vi "Get Environment Variable.vi"(7 "Target (Process)":T1 items=["Process", "User", "Machine"], 8 "Error In":errorcluster, 11 "Name":string) -> (0 "Error Out":errorcluster, 3 "Value":string)   [LabVIEW 2019, in "SLL Environment Variable.lvlib"]
doc: "Get <B>Value</B> of environment variable from <B>Target</B> environment."
uses:
  SLL Environment Variable.lvlib
  _Typedef/Target Environment Enum.ctl
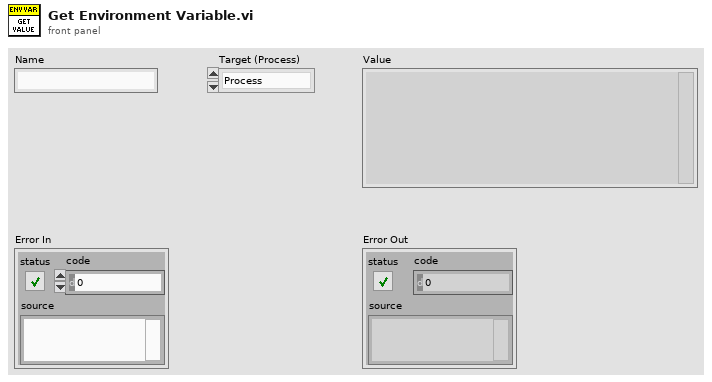
[diagram p1: front panel]
types:
  T1 = typedef "SLL Environment Variable.lvlib/Target Environment Enum.ctl" = i32
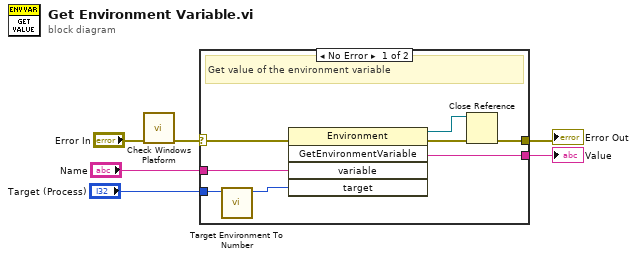
[diagram p0: block diagram]
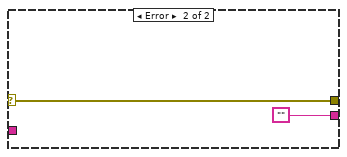
[diagram p2: hidden frame]
diagram:
  n1 = call "Check Windows Platform.vi"("Error In"="Error In") -> ("Error Out"=w2:errorcluster)  [unwired: 10 in]
  n2 = case shown="No Error" w2 {
    selector: w2 -> [w14 w16]
    tunnel: "Name" -> [w13 _]
    tunnel: [w11 ""] -> w5
    tunnel: [w10 w16] -> w4
    tunnel: "Target (Process)" -> [w8 _]
    frame No Error {
      # "Get value of the environment variable"
      n3 = call "Target Environment To Number.vi"("Target (Process)"=w8) -> ("Numeric Value"=w7:i32)  [unwired: 10 in]
      n4 = invoke class="Environment" method="GetEnvironmentVariable"(error in=w14, "variable"=w13, "target"=w7) -> (reference out=w9:refnum<k24>, error out=w12:errorcluster, "GetEnvironmentVariable"=w11:string)  [unwired: 2 in, 2 out]
      n5 = Close Reference(reference=w9, error in (no error)=w12) -> (error out=w10:errorcluster)
    }
    frame Error {
    }
  }
  "Error Out" <- w4
  "Value" <- w5
